vi "DTACQ - Download Data Block (Demultiplexed - Signed 16 Bit).vi"(8 "error in":errorcluster, 9 "Maximum Number of Samples":i32, 10 "Channel Number":i32, 11 "Address":string) -> (0 "error out":errorcluster, 1 "Data Overflow":bool, 2 "(Signed) 16 Bit Array":i16[](array[numeric]))   [LabVIEW 2017, in "Communications Library.lvlib"]
doc: "Downloads demultiplexed data from the DTACQ device, in 16 bit integer format, and returns the data."
uses:
  Communications Library.lvlib
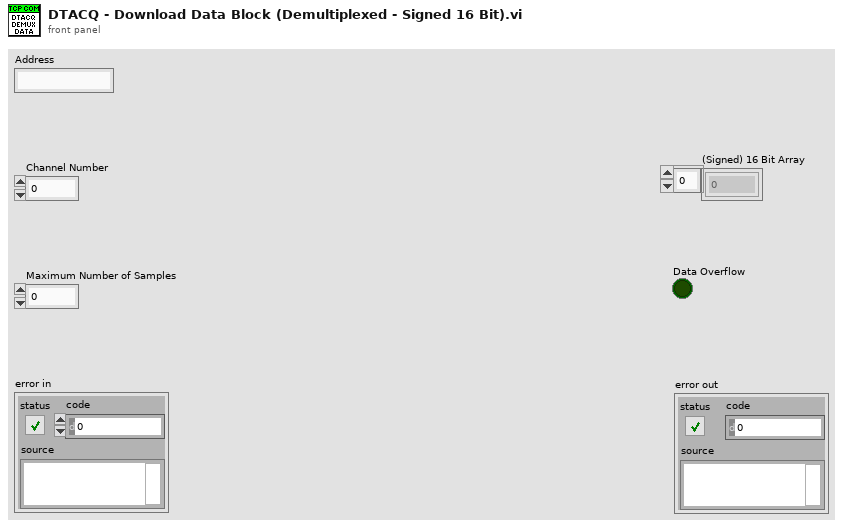
[diagram p1: front panel]
types:
  T1 = typedef "Communications Library.lvlib/DTACQ Connection Data--Cluster.ctl" = cluster{"Description":string, "Address":string, "Port":u16, "timeout (ms)":i32, "Termination Character":string, "TCP Connection Reference":refnum<k5>, "Open Connection":bool}
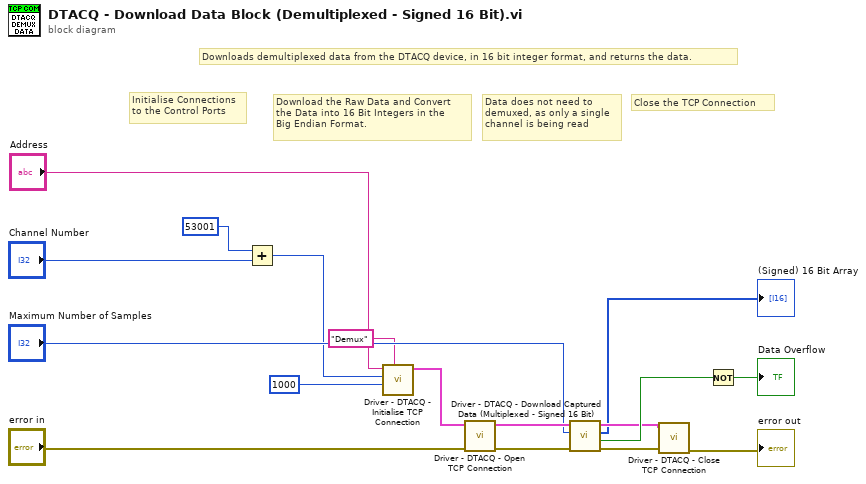
[diagram p0: block diagram]
diagram:
  # "Downloads demultiplexed data from the DTACQ device, in 16 bit integer format, and returns the data."
  # "Close the TCP Connection"
  # "Data does not need to\ndemuxed, as only a single\nchannel is being read"
  # "Download the Raw Data and Convert\nthe Data into 16 Bit Integers in the\nBig Endian Format."
  # "Initialise Connections\nto the Control Ports"
  n1 = Add(x=53001, y="Channel Number") -> (x+y=w4:i32)
  n2 = call "Driver - DTACQ - Initialise TCP Connection.vi"("Description"="Demux", "timeout (ms)"=1000, "Port"=w4, "Address"="Address") -> ("DTACQ Connection Data Out"=w14:T1)  [unwired: 7 in]
  n3 = call "Driver - DTACQ - Open TCP Connection.vi"("error in"="error in", "DTACQ Connection Data In"=w14) -> ("error out"=w15:errorcluster, "DTACQ Connection Data Out"=w12:T1)  [unwired: 8 in]
  n4 = call "Driver - DTACQ - Download Captured Data (Multiplexed - Signed 16 Bit).vi"("error in"=w15, "Samples"="Maximum Number of Samples", "DTACQ Connection Data In"=w12) -> ("error out"=w9:errorcluster, "Timed Out"=w17:bool, "(Signed) 16 Bit Array"=→"(Signed) 16 Bit Array":i16[], "DTACQ Connection Data Out"=w7:T1)  [unwired: 5 in]
  n5 = call "Driver - DTACQ - Close TCP Connection.vi"("error in"=w9, "DTACQ Connection Data In"=w7) -> ("error out"=→"error out":errorcluster)  [unwired: 8 in, 1 out]
  n6 = Not(x=w17) -> (.not. x?=→"Data Overflow":bool)
